vi "Serialize To Inputs.vi"(0 "Input 6":variant, 4 "Input 5":variant, 6 "Input 4":variant, 8 "Input 3":variant, 9 "Input 2":variant, 10 "Input 1":variant, 11 "TEMPLATE Event in":refnum<class "TEMPLATE Event.lvclass">) -> (3 "TEMPLATE Event out":refnum<class "TEMPLATE Event.lvclass">)   [LabVIEW 2021, in "_Template.lvlib" / "Templates.lvlib" / "TEMPLATE Event.lvlib" / "TEMPLATE Event.lvclass"]
uses:
  TEMPLATE Event.lvclass
  TEMPLATE Event.lvclass/TEMPLATE Event.ctl
  jettl/jettl/Event/Event.lvclass
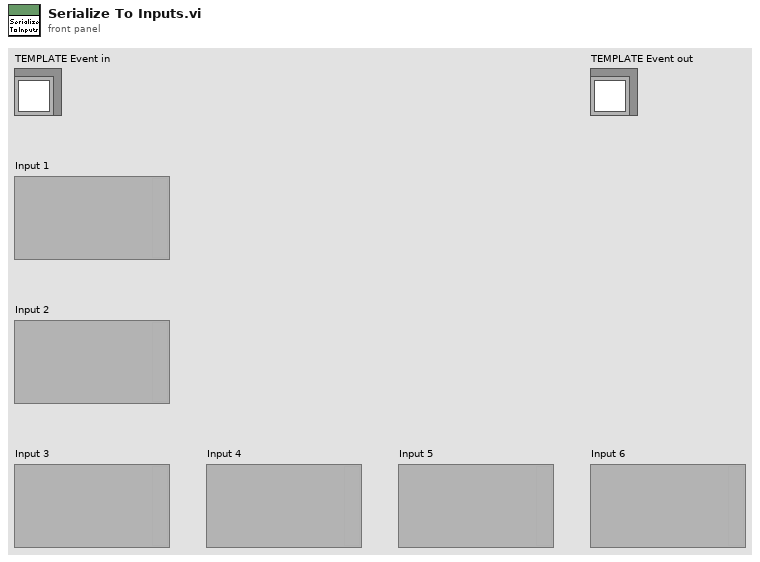
[diagram p1: front panel]
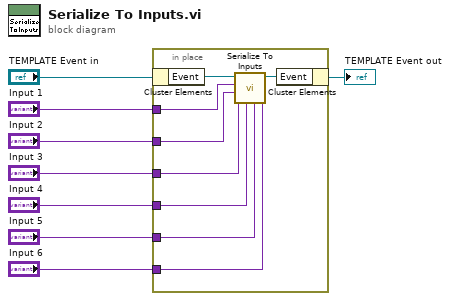
[diagram p0: block diagram]
diagram:
  n1 = in-place {
    in-place-border: "Input 1" -> [w14]
    in-place-border: "Input 2" -> [w13]
    in-place-border: "Input 3" -> [w12]
    in-place-border: "Input 4" -> [w11]
    in-place-border: "Input 5" -> [w10]
    in-place-border: "Input 6" -> [w9]
    n2 = in-place-cluster #1("TEMPLATE Event in") -> ("Event"=w16:refnum<class "Event.lvclass">)
    n3 = call-dynamic "Serialize To Inputs.vi"("Input 6"=w9, "Input 5"=w10, "Input 4"=w11, "Input 3"=w12, "Input 2"=w13, "Input 1"=w14, "jettl in"=w16) -> ("jettl out"=w15:refnum<class "Event.lvclass">)  [unwired: 4 in]
    n4 = in-place-cluster #1("Event"=w15) -> (→"TEMPLATE Event out":refnum<class "TEMPLATE Event.lvclass">)
  }
